vi "ClearClassNameCache.vi"(8 "error in (no error)":errorcluster, 11 "ClassName Cache":refnum<data-value>) -> (0 "error out":errorcluster, 3 "ClassName Cache":refnum<data-value>)   [LabVIEW 2019, in "BlueSerialization.lvlib" / "BlueSerializer.lvclass"]
uses:
  BlueSerializer.lvclass
  ClassNameCacheMap.ctl
  ClassNameObj.ctl
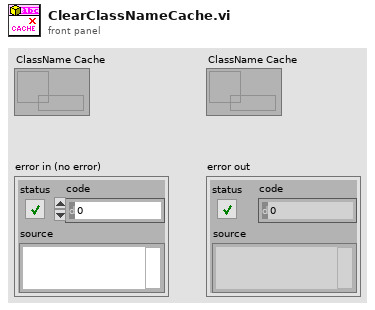
[diagram p1: front panel]
types:
  T1 = typedef "BlueSerialization.lvlib/BlueSerializer.lvclass/ClassNameCacheMap.ctl" = map{string, T2[]}
  T2 = typedef "BlueSerialization.lvlib/BlueSerializer.lvclass/ClassNameObj.ctl" = cluster{"class name":string, "default object":refnum<class>}
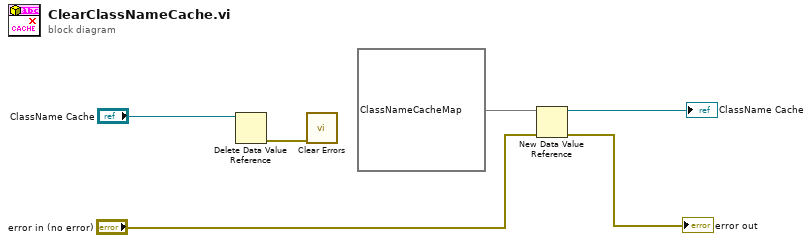
[diagram p0: block diagram]
diagram:
  n1 = Delete Data Value Reference(data value reference="ClassName Cache") -> (error out=w3:errorcluster)  [unwired: 1 in, 1 out]
  n2 = call <vilib>:"Clear Errors.vi"("error in (no error)"=w3) -> ()  [unwired: 5 in, 2 out]
  n3 = New Data Value Reference(data value=T1 {}, error in="error in (no error)") -> (data value reference=→"ClassName Cache":refnum<data-value>, error out=→"error out":errorcluster)
